vi "Untitled 4.vi"() -> ()   [LabVIEW 2018]
uses:
  <vilib>/robotics/Kinematics/DH Kinematic Parameters.ctl
  <vilib>/robotics/Kinematics/Link/Joint Type.ctl
  <vilib>/robotics/Kinematics/Analytical/Initialize Generic Serial Arm.vi
  <vilib>/robotics/Kinematics/Generate Cartesian Trajectory (Int).vi
  <vilib>/robotics/Kinematics/Robot/Inverse Kinematics (Point).vi
  <vilib>/robotics/Kinematics/Robot/Forward Kinematics (Point).vi
  <vilib>/picture/3D Picture Control/Object/Add Object (reference).vi
  <vilib>/robotics/Kinematics/NI_Kinematics.lvlib
  <vilib>/robotics/Kinematics/Plotting/NI_Robotics_3DKinematics.lvlib
  <vilib>/picture/3D Picture Control/NI_3D Picture Control.lvlib
  <vilib>/robotics/Kinematics/Analytical/NI_Robotics_AnalyticKinematics.lvlib
  <vilib>/robotics/Kinematics/Robot/NI_Robotics_Serial Robot Arm.lvclass
  <vilib>/robotics/Kinematics/Link/NI_Robotics_Link.lvclass
panel:
  out "joint positions 2":dbl[](array[numeric])
  in  "kinematic parameters 2":T1[](array[typedef])=[{"twist angle"=0.0, "length"=220.0, "rotation angle"=0.0, "offset distance"=20.85, "joint type"=enum."Revolute", "joint coordinate offset"=0.0}, {"twist angle"=0.0, "length"=200.0, "rotation angle"=0.0, "offset distance"=20.85, "joint type"=enum."Revolute", "joint coordinate offset"=0.0}, {"twist angle"=0.0, "length"=180.0, "rotation angle"=0.0, "offset distance"=20.85, "joint type"=enum."Revolute", "joint coordinate offset"=0.0}, {"twist angle"=0.0, "length"=0.0, "rotation angle"=0.0, "offset distance"=0.0, "joint type"=enum."Revolute", "joint coordinate offset"=0.0}]
  out "First Run Signal":bool=TRUE
  in  "Start X":dbl=-0.6
  in  "Start Y":dbl=-0.5
  in  "Start Z":dbl
  in  "End X":dbl
  in  "End Y":dbl=0.5
  in  "End Z":dbl=0.4
  out "Current X":dbl
  out "Current Y":dbl=0.5
  out "Current Z":dbl=0.4
  out "3D Picture Control":refnum<vi>(3d-picture)
  out "joint positions":dbl[](array[numeric])
  in  "Play":bool
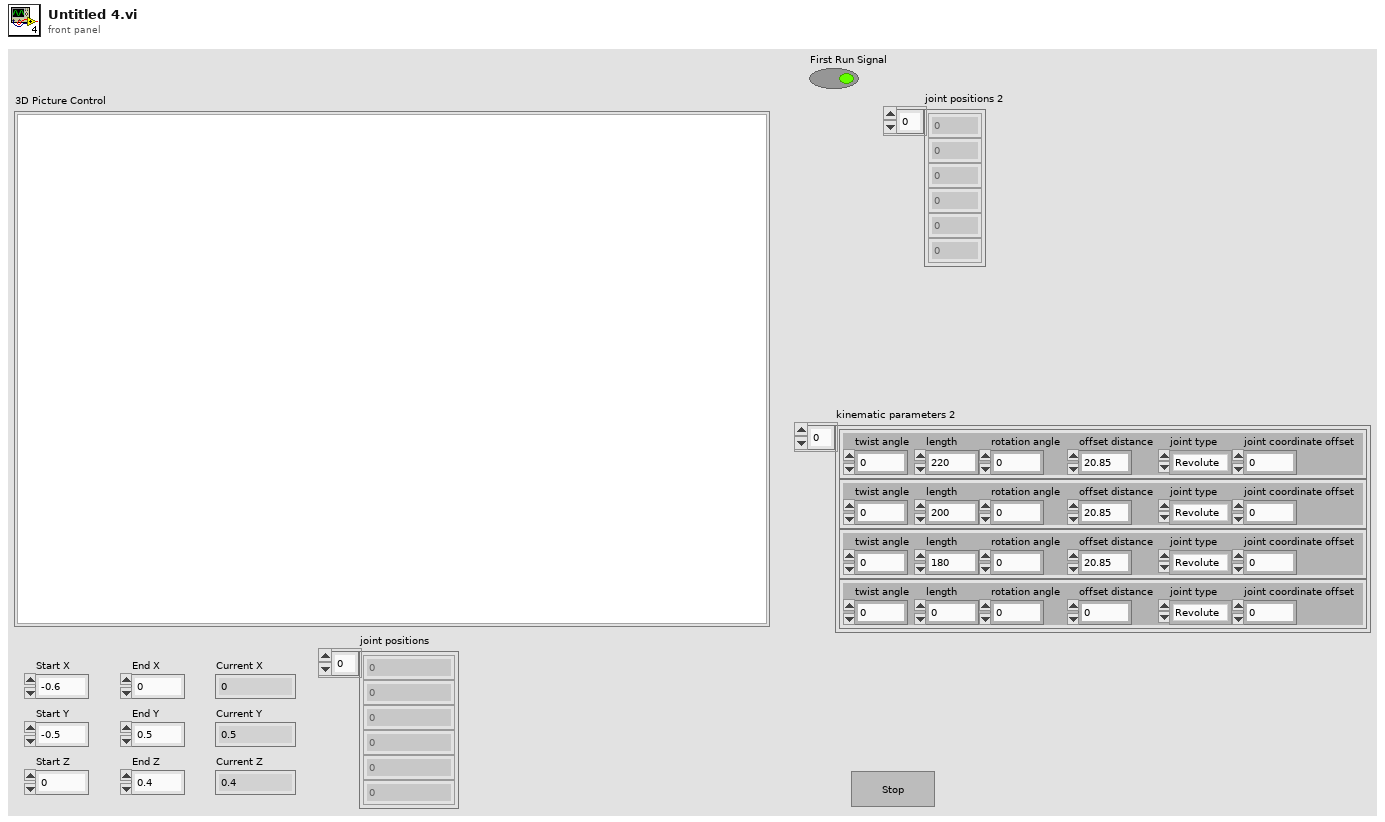
[diagram p1: front panel]
types:
  T1 = typedef "DH Kinematic Parameters.ctl" = cluster{"twist angle":dbl, "length":dbl, "rotation angle":dbl, "offset distance":dbl, "joint type":T2, "joint coordinate offset":dbl}
  T2 = typedef "NI_Robotics_Link.lvclass/Joint Type.ctl" = enum16{"Revolute", "Prismatic"}
  T3 = typedef "NI_Matrix.lvlib/RealMatrix.ctl" = dbl[][]
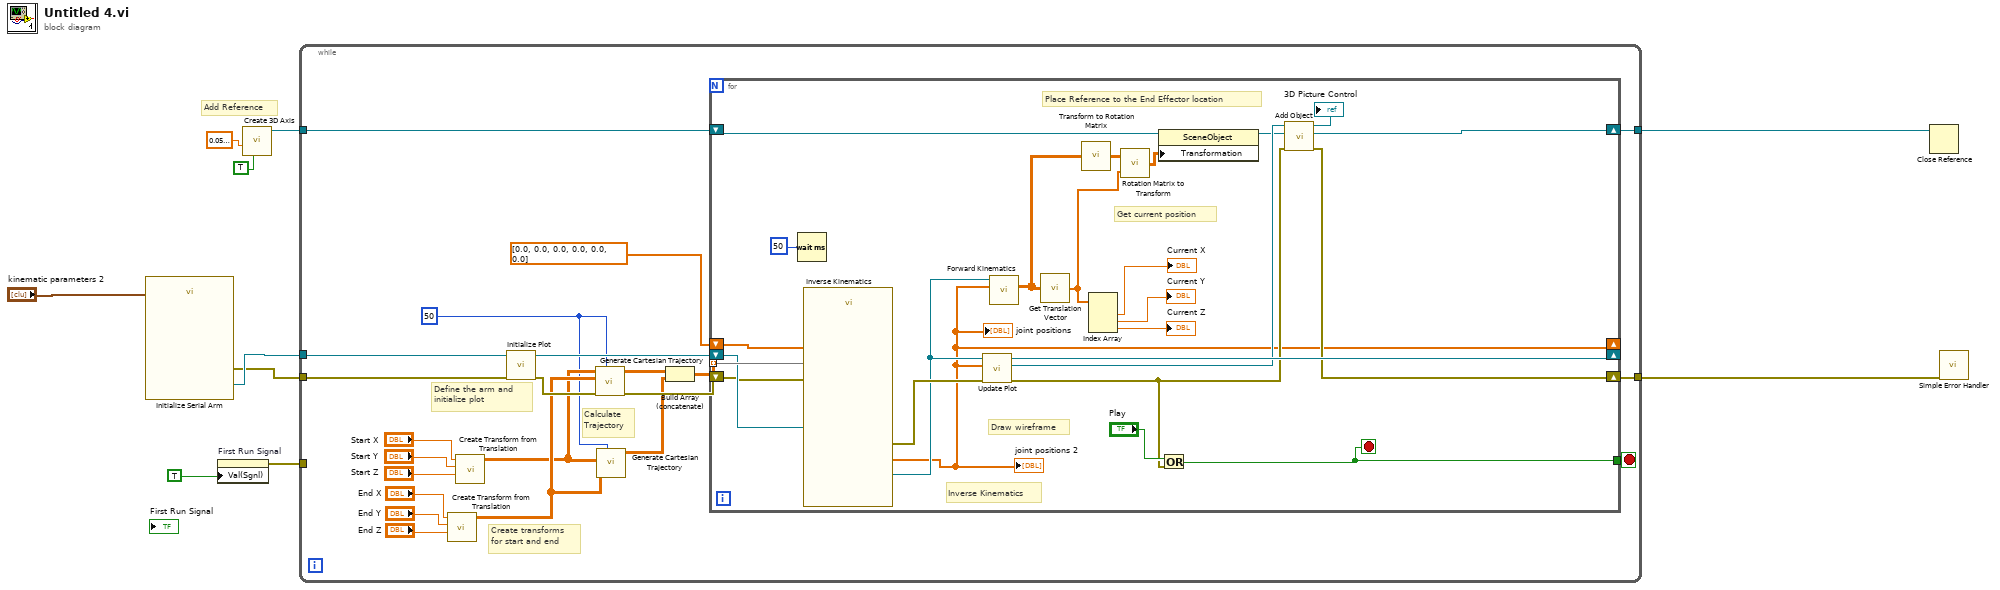
[diagram p0: block diagram]
diagram:
  # "Add Reference"
  n1 = call-poly <vilib>:"Initialize Serial Arm.vi"("kinematic parameters"="kinematic parameters 2") -> ("error out"=w2:errorcluster, "serial arm out"=w3:refnum<class "NI_Robotics_Serial Robot Arm.lvclass">)  [unwired: 9 in]
  n2 = property on="First Run Signal" class="Bool (strict)"("Val(Sgnl)"=TRUE ("Value (Signaling)")) -> (error out=w10:errorcluster)  [unwired: 2 in, 1 out]
  n3 = call <vilib>:"Create 3D Axis.vi"("Axis label?"=TRUE, "Radius"=sgl 0.05) -> ("New Object Refnum"=w6:refnum<vi>)  [unwired: 8 in, 1 out]
  n4 = while {
    tunnel: w10 -> [_]
    tunnel: w6 -> [w12]
    tunnel: [w22] -> w5
    tunnel: w3 -> [w16]
    tunnel: w2 -> [w15]
    tunnel: [w14] -> w4
    stop <- w13 stop-if-true
    w11 = 50
    # "Calculate \nTrajectory"
    # "Create transforms\nfor start and end"
    # "Define the arm and \ninitialize plot"
    n5 = call <vilib>:"Create Transform from Translation.vi"("z"="End Z", "y"="End Y", "x"="End X") -> ("transform"=w21:T3)  [unwired: 1 in, 7 out]
    n6 = call <vilib>:"Create Transform from Translation.vi"("z"="Start Z", "y"="Start Y", "x"="Start X") -> ("transform"=w20:T3)  [unwired: 1 in, 7 out]
    n7 = call <vilib>:"Initialize Plot.vi"("error in (no error)"=w15, "serial arm in"=w16) -> ("error out"=w25:errorcluster, "serial arm out"=w24:refnum<class "NI_Robotics_Serial Robot Arm.lvclass">)  [unwired: 8 in]
    n8 = call-poly <vilib>:"Generate Cartesian Trajectory.vi"("intermediate points"=w11, "error in (no error)"=w25, "end transform"=w21, "start transform"=w20) -> ("error out"=w26:errorcluster, "interpolated trajectory"=w19:dbl[][][])  [unwired: 6 in]
    n9 = call-poly <vilib>:"Generate Cartesian Trajectory.vi"("intermediate points"=w11, "end transform"=w20, "start transform"=w21) -> ("interpolated trajectory"=w17:dbl[][][])  [unwired: 7 in, 1 out]
    n10 = Build Array (concatenate)(w19, w17) -> (w18:dbl[][][])
    n11 = for {
      shift-right: [w36] -> w14
      shift-left: w26 -> [w53]
      tunnel: w18 -> [w56] mode=indexing
      shift-right: [w47] -> _
      shift-left: w24 -> [w55]
      shift-right: [w33] -> _
      shift-left: dbl[] [0.0, 0.0, 0.0, 0.0, 0.0, 0.0] ("joint positions") -> [w54]
      shift-right: [w40] -> w22
      shift-left: w12 -> [w42]
      tunnel: [w35] -> w13
      stop <- w35 stop-if-true
      # "Place Reference to the End Effector location"
      # "Get current position"
      # "Draw wireframe"
      # "Inverse Kinematics"
      n12 = Wait (ms)(milliseconds to wait=50) -> ()  [unwired: 1 out]
      n13 = call-poly <vilib>:"Inverse Kinematics.vi"("error in (no error)"=w53, "current joint positions"=w54, "end effector transform"=w56, "serial arm in"=w55) -> ("error out"=w49:errorcluster, "joint positions"=w33:dbl[], "serial arm out"=w48:refnum<class "NI_Robotics_Serial Robot Arm.lvclass">)  [unwired: 4 in, 1 out]
      "joint positions" <- w33
      "joint positions 2" <- w33
      n14 = call <vilib>:"Update Plot.vi"("error in (no error)"=w49, "joint positions"=w33, "serial arm in"=w48) -> ("error out"=w37:errorcluster, "serial arm scene"=w44:refnum<vi>, "serial arm out"=w47:refnum<class "NI_Robotics_Serial Robot Arm.lvclass">)  [unwired: 6 in]
      n15 = call-poly <vilib>:"Forward Kinematics.vi"("joint positions"=w33, "serial arm in"=w48) -> ("end effector transform"=w39:T3)  [unwired: 7 in, 2 out]
      n16 = call <vilib>:"Get Translation Vector.vi"("transform"=w39) -> ("translation vector"=w34:dbl[])
      n17 = call <vilib>:"Transform to Rotation Matrix.vi"("transform"=w39) -> ("rotation matrix"=w46:T3)
      n18 = Index Array(array=w34) -> (element #1=→"Current X":dbl, element #2=→"Current Y":dbl, element #3=→"Current Z":dbl)  [unwired: 3 in]
      n19 = call <vilib>:"Rotation Matrix to Transform.vi"("translation vector"=w34, "rotation matrix"=w46) -> ("transform"=w45:T3)
      n20 = property class="SceneObject"(reference=w42, "Transformation"=w45) -> (reference out=w41:refnum<vi>)  [unwired: 1 in, 1 out]
      n21 = Or(x="Play", y=w37) -> (x .or. y?=w35:bool)
      n22 = call-poly <vilib>:"Add Object.vi"("error in (no error)"=w37, "New Object In"=w41, "Scene Object In"=w44) -> ("error out"=w36:errorcluster, "New Object Out"=w40:refnum<vi>, "Scene Object Out"=→"3D Picture Control":refnum<vi>)  [unwired: 6 in]
    }
  }
  n23 = Close Reference(reference=w5) -> ()  [unwired: 1 in, 1 out]
  n24 = call <vilib>:"Simple Error Handler.vi"("error in (no error)"=w4) -> ()  [unwired: 4 in, 5 out]
